vi "MathCad_Easy_String_Set_Var.vi"(8 "error in (no error)":errorcluster, 9 "Variable Name":string, 10 "String Value":string, 11 "Mathcad Reference":T1) -> (0 "error out":errorcluster, 3 "Mathcad Reference":T1)   [LabVIEW 2015]
doc: "Sets numeric value in Mathcad. You can also use this VI to reset a variable that has already been set once. It is only dependent upon the variable name. The variable won't appear in the Mathcad worksheet, but is defined at the very beginning of the worksheet.\n\nInputs \n Wrksht Ref--ActiveX Reference to Mathcad Worksheet Class\n Value (String)--Value of Variable to Set\n New Variable Name(String)--Name of Variable to Set\n\nOutputs \n Wrksht Ref--ActiveX Reference to Mathcad Worksheet Class"
uses:
  Mathcad Reference.ctl
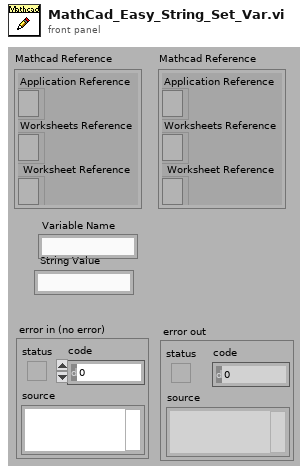
[diagram p1: front panel]
types:
  T1 = typedef "Mathcad Reference.ctl" = cluster{"Application Reference":refnum<k7>, "Worksheets Reference":refnum<k7>, " Worksheet Reference":refnum<k7>}
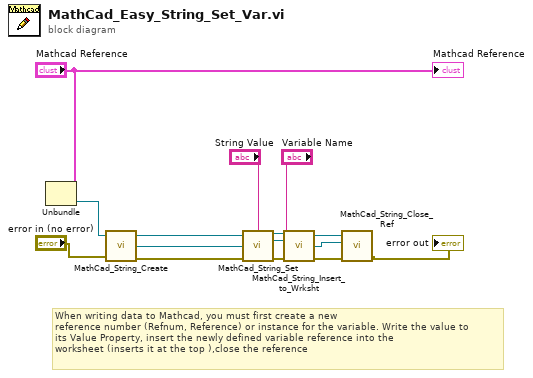
[diagram p0: block diagram]
diagram:
  # "When writing data to Mathcad, you must first create a new \nreference number (Refnum, Reference) or instance for the variable. Write the value to\nits Value Property, insert the newly defined variable reference into the\nworksheet (inserts it at the top ),close the reference"
  n1 = Unbundle("Mathcad Reference") -> ("Worksheet Reference"=w3:refnum<k7>)  [unwired: 2 out]
  n2 = call "MathCad_String_Create.vi"("error in (no error)"="error in (no error)", "Worksheet Reference In"=w3) -> ("error out"=w12:errorcluster, "Mathcad.IStringValue"=w13:refnum<k7>, "Worksheet Reference Out"=w14:refnum<k7>)  [unwired: 1 in]
  n3 = call "MathCad_String_Set.vi"("Worksheet Reference In"=w14, "value"="String Value", "Mathcad.IStringValue"=w13, "error in"=w12) -> ("Worksheet Reference Out"=w9:refnum<k7>, "Mathcad.IStringValue Out"=w8:refnum<k7>, "error out"=w7:errorcluster)  [unwired: 9 in]
  n4 = call "MathCad_String_Insert_to_Wrksht.vi"("error out 2"=w7, "New Variable Name"="Variable Name", "Mathcad.IStringValue"=w8, "Worksheet Reference In"=w9) -> ("error out"=w4:errorcluster, "Mathcad.IStringValue"=w11:refnum<k7>, "Worksheet Reference Out"=w10:refnum<k7>)
  n5 = call "MathCad_String_Close_Ref.vi"("error in"=w4, "Mathcad.IStringValue"=w11, "IMathcadWorksheet reference in"=w10) -> ("error out"=→"error out":errorcluster)  [unwired: 2 in, 1 out]
  "Mathcad Reference" <- "Mathcad Reference"
